vi "PH_Switch_USB.set GUI elements.vi"(0 "i ref in":refnum<vi>, 5 "error in (no error)":errorcluster) -> (14 "i ref out":refnum<vi>, 19 "error out":errorcluster)   [LabVIEW 2014, in "PH_Switch_USB.lvlib"]
doc: "Set GUI front panel elements depending on data base entries."
uses:
  PH_Switch_USB.lvlib
  PH_Basics/PH_Common/PH_Common.lvlib
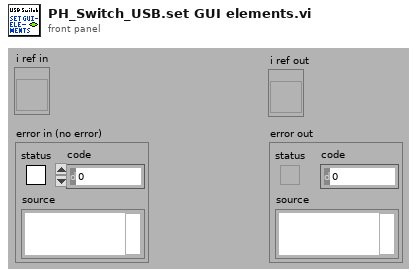
[diagram p1: front panel]
types:
  T1 = typedef "PH_Switch_USB.lvlib/PH_Switch_USB.i attribute.ctl" = cluster{"GUI Refs":cluster{"GUI-Knob":refnum<vi>, "Delete":refnum<vi>}, "Switch":cluster{"GUI Ref":refnum<vi>, "Service name":string, "Array No.":i16, "caption":string, "Status":T2}, "True-Sensor":cluster{"GUI Ref":refnum<vi>, "Service name":string, "Array No.":i16, "caption":string, "Status":T2}, "False-Sensor":cluster{"GUI Ref":refnum<vi>, "Service name":string, "Array No.":i16, "caption":string, "Status":T2}}
  T2 = typedef "PH_StatusHandler.lvlib/PH_StatusHandler.Status.ctl" = i16
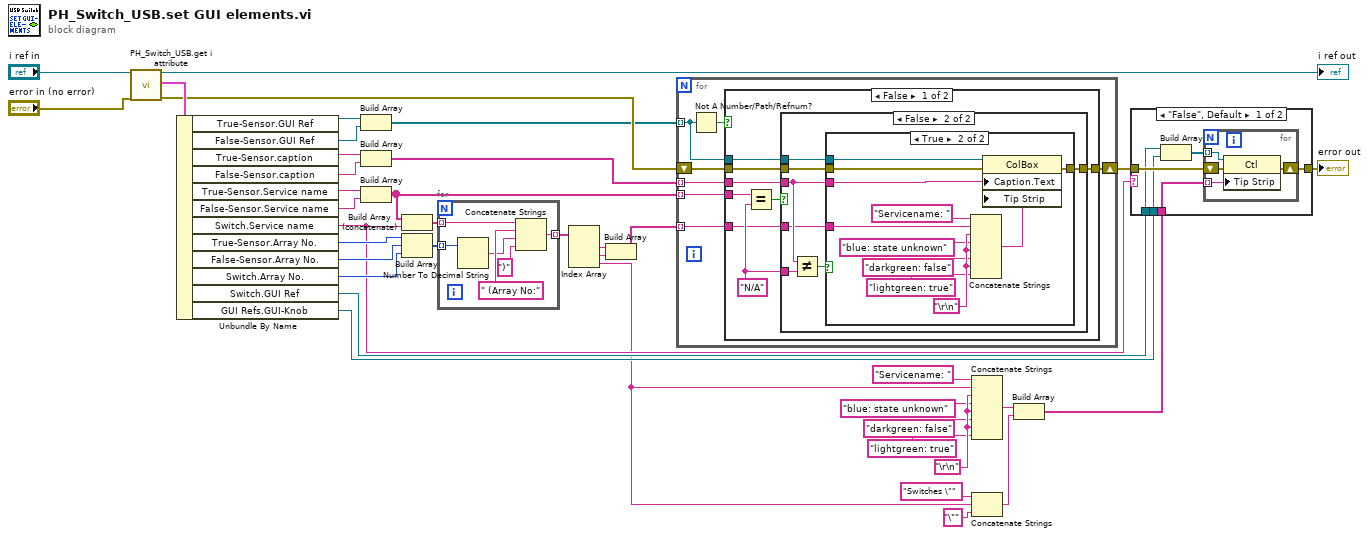
[diagram p0: block diagram]
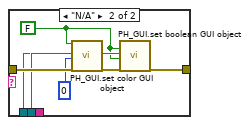
[diagram p2: hidden frame]
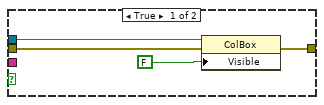
[diagram p3: hidden frame]
diagram:
  w22 = "\r\n"
  n1 = call "PH_Switch_USB.get i attribute.vi"("i ref in"="i ref in", "error in (no error)"="error in (no error)") -> ("i ref out"=→"i ref out":refnum<vi>, "i attribute"=w39:T1, "error out"=w35:errorcluster)  [unwired: 15 in]
  n2 = Unbundle By Name(w39) -> ("True-Sensor.GUI Ref"=w34:refnum<vi>, "False-Sensor.GUI Ref"=w33:refnum<vi>, "True-Sensor.caption"=w31:string, "False-Sensor.caption"=w30:string, "True-Sensor.Service name"=w32:string, "False-Sensor.Service name"=w13:string, "Switch.Service name"=w5:string, "True-Sensor.Array No."=w11:i16, "False-Sensor.Array No."=w10:i16, "Switch.Array No."=w9:i16, "Switch.GUI Ref"=w25:refnum<vi>, "GUI Refs.GUI-Knob"=w24:refnum<vi>)
  n3 = Build Array(w34, w33) -> (w29:refnum<vi>[])
  n4 = Build Array(w31, w30) -> (w28:string[])
  n5 = Build Array(w32, w13) -> (w12:string[])
  n6 = Build Array (concatenate)(w12, w5) -> (w7:string[])
  n7 = Build Array(w11, w10, w9) -> (w8:i16[])
  n8 = for {
    tunnel: w8 -> [w45] mode=indexing
    tunnel: w7 -> [w44] mode=indexing
    tunnel: [w40] -> w6 mode=indexing
    n9 = Number To Decimal String(number=w45) -> (decimal integer string=w42:string)  [unwired: 1 in]
    n10 = Concatenate Strings(w44, " (Array No:" ("string"), w42, ")" ("string")) -> (w40:string)
  }
  n11 = Index Array(array=w6) -> (element #1=w3:string, element #2=w2:string, element #3=w4:string)  [unwired: 3 in]
  n12 = Build Array(w3, w2) -> (w1:string[])
  n13 = for {
    tunnel: w28 -> [w52] mode=indexing
    tunnel: w29 -> [w50] mode=indexing
    tunnel: w12 -> [w48] mode=indexing
    shift-right: [w47] -> w26
    shift-left: w35 -> [w49]
    tunnel: w1 -> [w46] mode=indexing
    n14 = Not A Number/Path/Refnum?(number/path/refnum=w50) -> (NaN/Path/Refnum?=w51:bool)
    n15 = case shown="False" w51 {
      tunnel: w52 -> [w60 _]
      tunnel: w48 -> [w54 _]
      tunnel: [w58 w84] -> w47
      tunnel: w49 -> [w57 w84]
      tunnel: w50 -> [w56 _]
      tunnel: w46 -> [w53 _]
      frame False {
        w55 = "N/A" ("x")
        n16 = Equal?(x=w54, y=w55) -> (x = y?=w59:bool)
        n17 = case shown="False" w59 {
          tunnel: w56 -> [w64 w71]
          tunnel: w57 -> [w63 w70]
          tunnel: [w62 w69] -> w58
          tunnel: w60 -> [_ w66]
          tunnel: w55 -> [_ w67]
          tunnel: w53 -> [_ w65]
          frame True {
            n18 = property class="ColBox"(reference=w64, error in=w63, "Visible"=FALSE) -> (error out=w62:errorcluster)  [unwired: 1 out]
          }
          frame False {
            n19 = Not Equal?(x=w66, y=w67) -> (x != y?=w68:bool)
            n20 = case shown="True" w68 {
              tunnel: w71 -> [_ w83]
              tunnel: w70 -> [w72 w82]
              tunnel: [w72 w81] -> w69
              tunnel: w66 -> [_ w80]
              tunnel: w65 -> [_ w74]
              frame False {
              }
              frame True {
                w78 = "\r\n"
                n21 = Concatenate Strings("Servicename: ", w74, w78, "blue: state unknown", w78, "darkgreen: false", w78, "lightgreen: true") -> (w73:string)
                n22 = property class="ColBox"(reference=w83, error in=w82, "Caption.Text"=w80, "Tip Strip"=w73) -> (error out=w81:errorcluster)  [unwired: 1 out]
              }
            }
          }
        }
      }
      frame True {
      }
    }
  }
  n23 = Concatenate Strings("Servicename: ", w4, w22, "blue: state unknown", w22, "darkgreen: false", w22, "lightgreen: true") -> (w16:string)
  n24 = Concatenate Strings("Switches \"" ("string"), w4, "\"" ("string")) -> (w15:string)
  n25 = Build Array(w16, w15) -> (w14:string[])
  n26 = case shown="\"False\", Default" w5 {
    tunnel: [w89 w100] -> w27
    tunnel: w26 -> [w90 w99]
    tunnel: w24 -> [w87 w98]
    tunnel: w25 -> [w88 w97]
    tunnel: w14 -> [w85 _]
    frame "False", Default {
      n27 = Build Array(w88, w87) -> (w86:refnum<vi>[])
      n28 = for {
        tunnel: w86 -> [w92] mode=indexing
        shift-right: [w93] -> w89
        shift-left: w90 -> [w94]
        tunnel: w85 -> [w91] mode=indexing
        n29 = property class="Ctl"(reference=w92, error in=w94, "Tip Strip"=w91) -> (error out=w93:errorcluster)  [unwired: 1 out]
      }
    }
    frame "N/A" {
      w96 = FALSE ("Value")
      n30 = call "PH_GUI.set color GUI object.vi"("Visible? (true)"=w96, "GUI object Ref"=w97, "State"=0, "error in (no error)"=w99) -> ("error out"=w101:errorcluster)  [unwired: 15 in]
      n31 = call "PH_GUI.set boolean GUI object.vi"("Visible (true)"=w96, "Boolean Knob GUI Ref"=w98, "Value"=w96, "error in (no error)"=w101) -> ("error out"=w100:errorcluster)  [unwired: 15 in]
    }
  }
  "error out" <- w27
